vi "Client Generator Error Strings Global.vi"() -> ()   [LabVIEW 2021, in "MeasurementClient Editor.lvlib"]
uses:
  MeasurementClient Editor.lvlib
panel:
  out "5101":string="Measurements with no configuration or results are not supported by the tool."
  out "5100":string="Internal error. No case found for the control name '%s'."
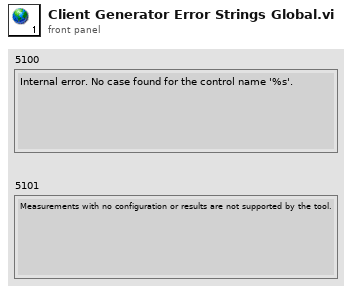
[diagram p1: front panel]
diagram:
